vi "prop_graph_main.vi"() -> ()   [LabVIEW 2020, in "3DPC_SurfacePlot.xctl"]
uses:
  <vilib>/Native 3D Graph/xcontrol/3DPC_SurfacePlot.xctl
  <vilib>/Native 3D Graph/typedefs/prop_graph.ctl
  <vilib>/Utility/miscctls.llb/LVPointTypeDef.ctl
panel:
  in  "done":refnum<user-event>
  in  "quit":refnum<user-event>
  out "Graph Properties Out":T1
  in  "Graph Properties In":T1
  in  "Tab Graph Prop":enum32{"General", "3D", "Grid Planes"}(tab)
  in  "Lighting":bool
  in  "Plot Area Color":u32(colorbox)
  in  "Fast Draw":bool caption="Fast Draw For\nPan/Zoom/Rotate"
  in  "Projection Enum":u16(ring) caption="Projection" items=["Orthographic", "Perspective"]
  in  "View Direction":T2(radio)
  in  "X-Z":bool
  in  "Y-Z":bool
  in  "X-Y":bool
  # "Show Grid Planes"
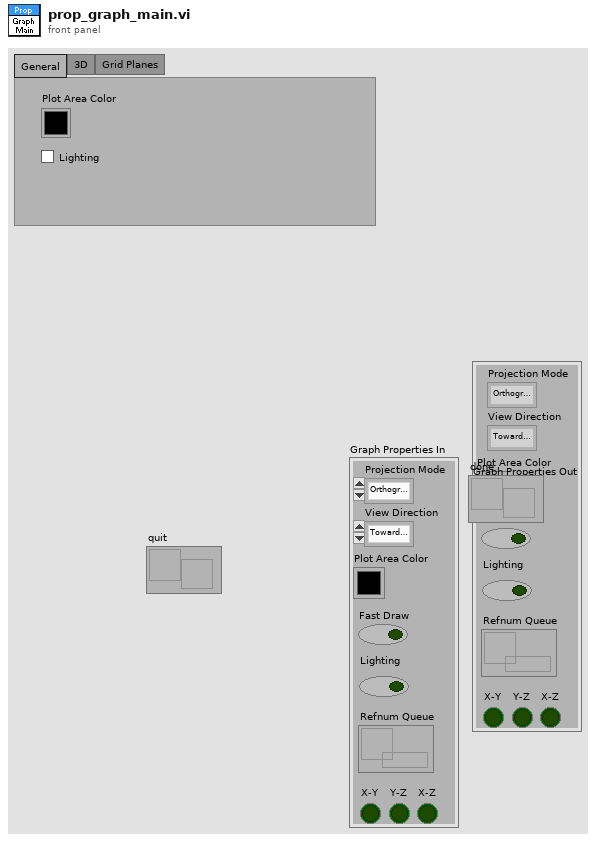
[diagram p1: front panel]
types:
  T1 = typedef "3DPC_SurfacePlot.xctl/prop_graph.ctl" = cluster{"Projection Mode":enum16{"Orthographic", "Perspective"}, "View Direction":enum32{"Towards X-Y Plane", "Towards Y-Z Plane", "Towards X-Z Plane", "User Define"}, "Plot Area Color":u32, "Fast Draw":bool, "X-Y":bool, "Y-Z":bool, "X-Z":bool, "Lighting":bool, "Refnum Queue":refnum<queue>}
  T2 = enum32{"Towards X-Y Plane", "Towards Y-Z Plane", "Towards X-Z Plane", "User Define"}
  T3 = typedef "LVPointTypeDef.ctl" = cluster{"Horizontal":i16, "Vertical":i16}
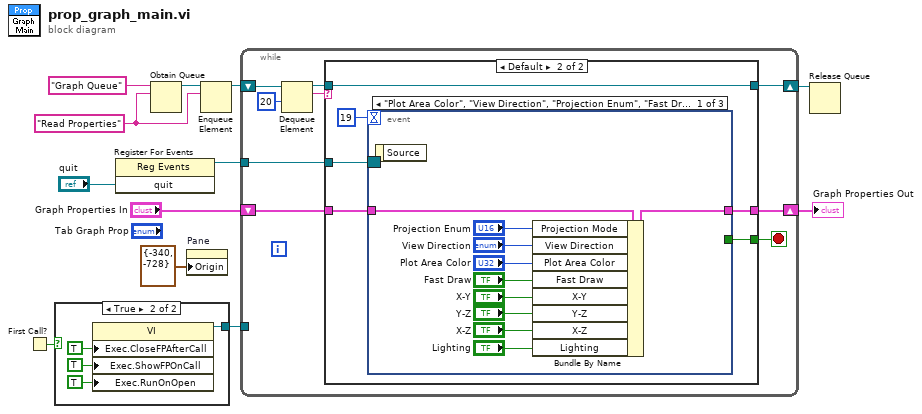
[diagram p0: block diagram]
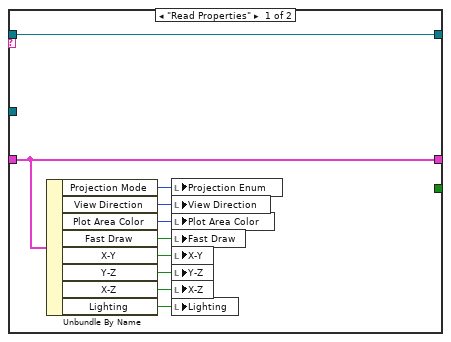
[diagram p3: hidden frame]
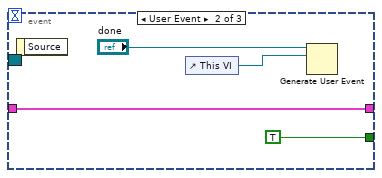
[diagram p4: hidden frame]
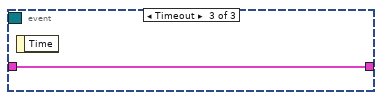
[diagram p5: hidden frame]
diagram:
  w10 = "Read Properties"
  n1 = First Call?() -> (First Call?: T/F=w1:bool)
  n2 = case shown="True" w1 {
    tunnel: [_ w14] -> w7
    frame False {
    }
    frame True {
      n3 = property class="VI"("Exec.CloseFPAfterCall"=TRUE ("Execution:Close After Call"), "Exec.ShowFPOnCall"=TRUE ("Execution:Show Front Panel On Call"), "Exec.RunOnOpen"=TRUE ("Execution:Run When Opened")) -> (reference out=w14:refnum<vi>)  [unwired: 2 in, 1 out]
    }
  }
  n4 = register-events("quit") -> (reference out=w3:refnum<event-registration>)  [unwired: 2 in, 1 out]
  n5 = Obtain Queue(name (unnamed)="Graph Queue", element data type=w10) -> (queue out=w11:refnum<queue>)  [unwired: 3 in, 2 out]
  n6 = property on="Pane" class="Pane"("Origin"=T3 {"Horizontal"=-340, "Vertical"=-728} ("Point")) -> ()  [unwired: 2 in, 2 out]
  n7 = Enqueue Element(queue=w11, element=w10) -> (queue out=w9:refnum<queue>)  [unwired: 1 in, 3 out]
  n8 = while {
    shift-right: [w21] -> w8
    shift-left: w9 -> [w24]
    tunnel: w7 -> [_]
    shift-right: [w19] -> w5
    shift-left: "Graph Properties In" -> [w20]
    tunnel: w3 -> [w18]
    stop <- w17 stop-if-true
    n9 = Dequeue Element(queue=w24, timeout in ms (-1)=20) -> (queue out=w22:refnum<queue>, element=w23:string)  [unwired: 1 in, 2 out]
    n10 = case shown="Default" w23 {
      tunnel: w22 -> [w35 w38]
      tunnel: [_ w36] -> w17
      tunnel: [w35 w38] -> w21
      tunnel: w20 -> [w30 w40]
      tunnel: [w30 w39] -> w19
      tunnel: w18 -> [_ w37]
      frame "Read Properties" {
        n11 = Unbundle By Name(w30) -> ("Projection Mode"=w31:enum16{"Orthographic", "Perspective"}, "View Direction"=w32:T2, "Plot Area Color"=w33:u32, "Fast Draw"=w34:bool, "X-Y"=w28:bool, "Y-Z"=w27:bool, "X-Z"=w29:bool, "Lighting"=w26:bool)
        n12 = local write "Projection Enum"(w31) -> ()
        n13 = local write "View Direction"(w32) -> ()
        n14 = local write "Plot Area Color"(w33) -> ()
        n15 = local write "Fast Draw"(w34) -> ()
        n16 = local write "X-Y"(w28) -> ()
        n17 = local write "Y-Z"(w27) -> ()
        n18 = local write "X-Z"(w29) -> ()
        n19 = local write "Lighting"(w26) -> ()
      }
      frame Default {
        n20 = event shown="[0] \"Plot Area Color\", \"View Direction\", \"Projection Enum\", \"Fast Draw\", \"X-Y\", \"Y-Z\", \"X-Z\", \"Lighting\": Value Change" {
          selector: w37 -> [_ _ _]
          dyn-events: _ -> [_ _ _]
          timeout: 19 -> [_ _ _]
          tunnel: w40 -> [w51 w52 w56]
          tunnel: [w46 w52 w56] -> w39
          tunnel: [_ TRUE _] -> w36
          event "Plot Area Color", "View Direction", "Projection Enum", "Fast Draw", "X-Y", "Y-Z", "X-Z", "Lighting": Value Change {
            n21 = event-data() -> ()  [unwired: 2 out]
            n22 = Bundle By Name(cluster=w51, "Projection Mode"="Projection Enum", "View Direction"="View Direction", "Plot Area Color"="Plot Area Color", "Fast Draw"="Fast Draw", "X-Y"="X-Y", "Y-Z"="Y-Z", "X-Z"="X-Z", "Lighting"="Lighting") -> (w46:T1)
          }
          event User Event {
            n23 = event-data() -> ()  [unwired: 2 out]
            n24 = control-ref of="This VI"() -> (w54:refnum<vi>)
            n25 = Generate User Event(user event="done", event data cluster=w54) -> ()  [unwired: 2 in, 2 out]
          }
          event Timeout {
            n26 = event-data() -> ()  [unwired: 2 out]
          }
        }
      }
    }
  }
  "Graph Properties Out" <- w5
  n27 = Release Queue(queue=w8) -> ()  [unwired: 1 in, 4 out]
